vi "Layout.vi"(0 "FSM.Label In":refnum<class "FSM.Label.lvclass">) -> (4 "FSM.Label Out":refnum<class "FSM.Label.lvclass">)   [LabVIEW 2020, in "FSM.Label.lvclass"]
uses:
  FSM.Label.lvclass
  FSM.Label.lvclass/FSM.Label.ctl
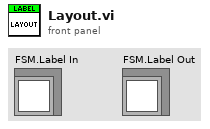
[diagram p1: front panel]
types:
  T1 = cluster{"horizontal":enum16{"left", "center", "right"}, "vertical":enum16{"top", "center", "bottom"}}
  T2 = cluster{"Font Name:":string, "Size":i16, "Strikeout?":bool, "Italic?":bool, "Underline?":bool, "Outline?":bool, "Shadow?":bool, "Bold?":bool}
  T3 = cluster{"left":i16, "top":i16, "right":i16, "bottom":i16}
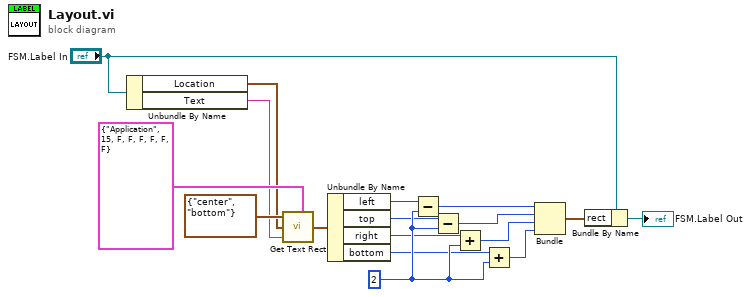
[diagram p0: block diagram]
diagram:
  w13 = 2
  n1 = Unbundle By Name("FSM.Label In") -> ("Location"=w4:cluster{"x":i16, "y":i16}, "Text"=w5:string)
  n2 = call <vilib>:"Get Text Rect.vi"("alignment(left, top)"=T1 {"horizontal"=enum."center", "vertical"=enum."bottom"}, "origin(0,0)"=w4, "text"=w5, "[user-specified font]"=T2 {"Font Name:"="Application", "Size"=15, "Strikeout?"=FALSE, "Italic?"=FALSE, "Underline?"=FALSE, "Outline?"=FALSE, "Shadow?"=FALSE, "Bold?"=FALSE}) -> ("rect"=w8:T3)  [unwired: 5 in]
  n3 = Unbundle By Name(w8) -> ("left"=w9:i16, "top"=w10:i16, "right"=w11:i16, "bottom"=w12:i16)
  n4 = Subtract(x=w9, y=w13) -> (x-y=w14:i32)
  n5 = Subtract(x=w10, y=w13) -> (x-y=w15:i32)
  n6 = Add(x=w11, y=w13) -> (x+y=w16:i32)
  n7 = Add(x=w12, y=w13) -> (x+y=w17:i32)
  n8 = Bundle(w14, w15, w16, w17) -> (w2:cluster{i32, i32, i32, i32})  [unwired: 1 in]
  n9 = Bundle By Name(cluster="FSM.Label In", "rect"=w2) -> (→"FSM.Label Out":refnum<class "FSM.Label.lvclass">)
